vi "write_ini_of_article.vi"(8 "Current Article":string, 9 "Current OF":string, 11 "Path_bench":path) -> ()   [LabVIEW 2014]
uses:
  <vilib>/Utility/config.llb/Write Key (String).vi
  <vilib>/Utility/config.llb/NI_LVConfig.lvlib
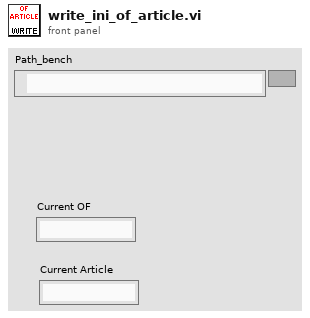
[diagram p1: front panel]
types:
  T1 = typedef "NI_LVConfig.lvlib/Config Data RefNum.ctl" = refnum<k1>
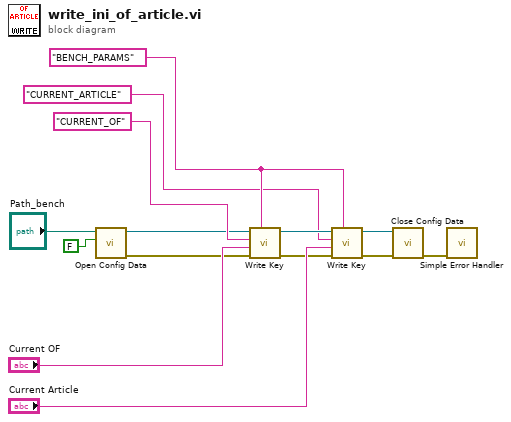
[diagram p0: block diagram]
diagram:
  w7 = "BENCH_PARAMS" ("section")
  n1 = call <vilib>:"Open Config Data.vi"("create file if necessary (T)"=FALSE, "configuration file path"="Path_bench") -> ("error out"=w3:errorcluster, "refnum"=w4:T1)  [unwired: 7 in, 1 out]
  n2 = call-poly <vilib>:"Write Key.vi"("section"=w7, "error in (no error)"=w3, "value"="Current OF", "key"="CURRENT_OF" ("Key 3"), "refnum"=w4) -> ("error out"=w2:errorcluster, "refnum out"=w11:T1)  [unwired: 4 in, 1 out]
  n3 = call-poly <vilib>:"Write Key.vi"("section"=w7, "error in (no error)"=w2, "value"="Current Article", "key"="CURRENT_ARTICLE" ("Key 3"), "refnum"=w11) -> ("error out"=w1:errorcluster, "refnum out"=w10:T1)  [unwired: 4 in, 1 out]
  n4 = call <vilib>:"Close Config Data.vi"("error in (no error)"=w1, "refnum"=w10) -> ("error out"=w13:errorcluster)  [unwired: 8 in, 1 out]
  n5 = call <vilib>:"Simple Error Handler.vi"("error in (no error)"=w13) -> ()  [unwired: 4 in, 5 out]
